vi "message.vi"() -> ()   [LabVIEW 2022 SP3]
uses:
  LABVIEW FILE'S/comman 2.o.vi
panel:
  out "String":string
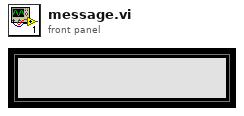
[diagram p1: front panel]
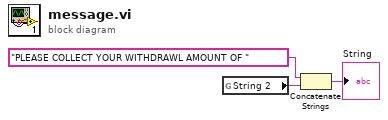
[diagram p0: block diagram]
diagram:
  n1 = global read "comman 2.o.vi" "String 2"() -> (w3:string)
  n2 = Concatenate Strings("PLEASE COLLECT YOUR WITHDRAWL AMOUNT OF " ("String"), w3) -> (→"String":string)
